vi "receive_photon_buffer.vi"(8 "error in (no error)":errorcluster, 11 "picoharp in":refnum<class "picoharp.lvclass">) -> (0 "error out":errorcluster, 2 "done":bool, 3 "picoharp out":refnum<class "picoharp.lvclass">)   [LabVIEW 2015, in "picoharp.lvclass"]
uses:
  picoharp.lvclass
  picoharp.lvclass/picoharp.ctl
  Hydraharp/hydraharp/hydraharp_fifo_queue_data.ctl
  Hydraharp/hydraharp/hydraharp_fifo_actions.ctl
  phlib.dll
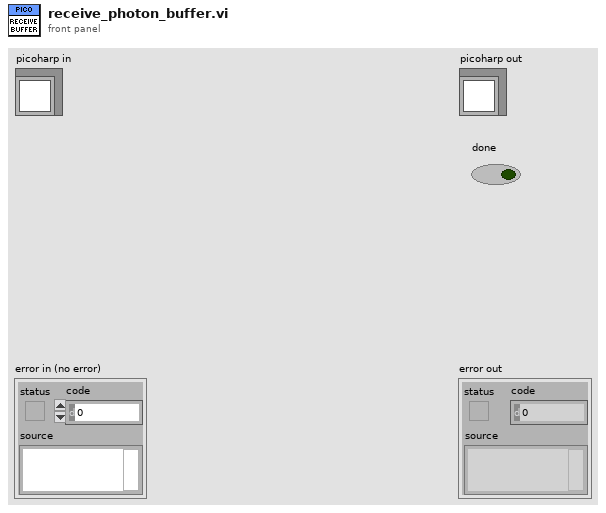
[diagram p1: front panel]
types:
  T1 = typedef "hydraharp_fifo_queue_data.ctl" = cluster{"fifo_buffer":u32[], "fifo_action":T2}
  T2 = typedef "hydraharp_fifo_actions.ctl" = enum16{"stop", "new_data"}
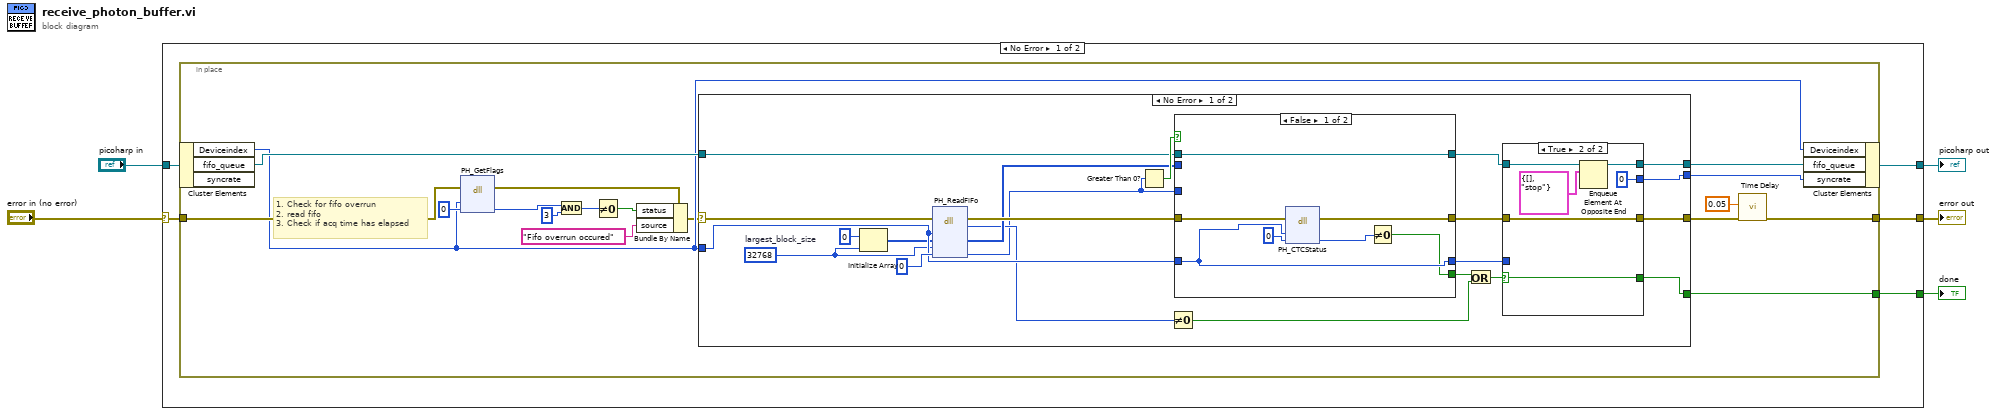
[diagram p0: block diagram]
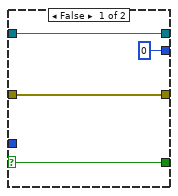
[diagram p2: hidden frame]
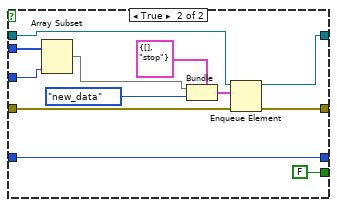
[diagram p3: hidden frame]
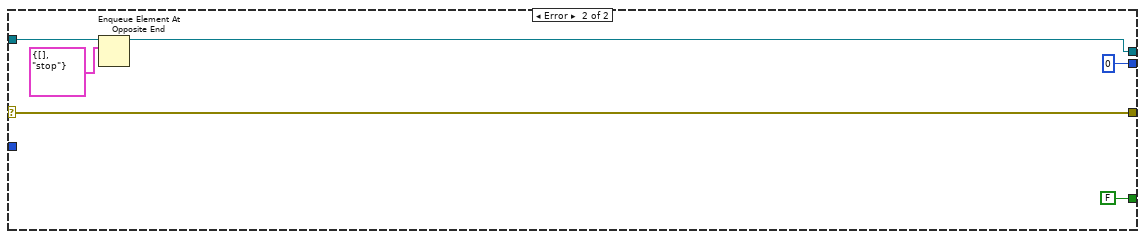
[diagram p4: hidden frame]
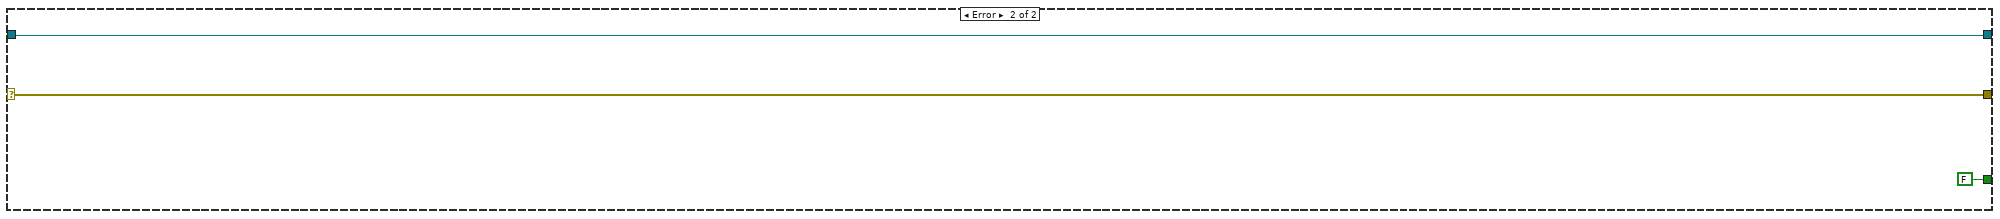
[diagram p5: hidden frame]
diagram:
  n1 = case shown="No Error" "error in (no error)" {
    selector: "error in (no error)" -> [w9 w87]
    tunnel: [w8 w87] -> w2
    tunnel: [w7 w86] -> w1
    tunnel: "picoharp in" -> [w10 w86]
    tunnel: [w6 FALSE] -> w3
    frame No Error {
      n2 = in-place {
        in-place-border: w9 -> [w27]
        in-place-border: [w12] -> w8
        in-place-border: [w20] -> w6
        # "1. Check for fifo overrun\n2. read fifo\n3. Check if acq time has elapsed"
        n3 = in-place-cluster #1(w10) -> ("Deviceindex"=w21:i32, "fifo_queue"=w23:refnum<queue>)  [unwired: 1 out]
        n4 = dll-call lib="phlib.dll" fn="PH_GetFlags" label="pH_GetFlags"(error in=w27, "devidx"=w21, "flags"=0) -> (error out=w19:errorcluster, "flags"=w25:i32)  [unwired: 4 in, 1 out]
        n5 = And(x=w25, y=3) -> (x .and. y?=w16:i32)
        n6 = Not Equal To 0?(x=w16) -> (x != 0?=w15:bool)
        n7 = Bundle By Name(cluster=w19, "status"=w15, "source"="Fifo overrun occured") -> (w17:errorcluster)
        n8 = case shown="No Error" w17 {
          selector: w17 -> [w37 w80]
          tunnel: w21 -> [w46 _]
          tunnel: w23 -> [w44 w84]
          tunnel: [w40 w83] -> w22
          tunnel: [w39 w80] -> w13
          tunnel: [w38 FALSE] -> w20
          tunnel: [w28 0 ("syncrate")] -> w11
          frame No Error {
            w31 = 32768  # largest_block_size
            n9 = Initialize Array(u32 0 ("element"), w31) -> (w30:u32[])
            n10 = dll-call lib="phlib.dll" fn="PH_ReadFiFo" label="pH_ReadFiFo"(error in=w37, "devidx"=w46, "buffer"=w30, "blocksize"=w31, "nactual"=0) -> (error out=w47:errorcluster, "return type"=w36:i32, "buffer"=w43:u32[], "nactual"=w33:i32)  [unwired: 4 in, 1 out]
            n11 = Greater Than 0?(x=w33) -> (x > 0?=w48:bool)
            n12 = Not Equal To 0?(x=w36) -> (x != 0?=w35:bool)
            n13 = case shown="False" w48 {
              tunnel: w47 -> [w66 w76]
              tunnel: [w65 w71] -> w34
              tunnel: w46 -> [w63 w67]
              tunnel: [w60 FALSE] -> w45
              tunnel: w44 -> [w64 w77]
              tunnel: w43 -> [_ w70]
              tunnel: [w64 w72] -> w41
              tunnel: w33 -> [_ w68]
              tunnel: [w63 w67] -> w29
              frame False {
                n14 = dll-call lib="phlib.dll" fn="PH_CTCStatus" label="pH_CTCStatus"(error in=w66, "devidx"=w63, "status"=0) -> (error out=w65:errorcluster, "status"=w61:i32)  [unwired: 4 in, 1 out]
                n15 = Not Equal To 0?(x=w61) -> (x != 0?=w60:bool)
              }
              frame True {
                n16 = Array Subset(array=w70, length=w68) -> (w69:u32[])  [unwired: 1 in]
                n17 = Bundle(cluster=T1 {"fifo_buffer"=[], "fifo_action"=enum."stop"} ("output cluster"), "fifo_buffer"=w69, "fifo_action"=hydraharp_fifo_actions."new_data") -> (w73:T1)
                n18 = Enqueue Element(queue=w77, element=w73, error in (no error)=w76) -> (queue out=w72:refnum<queue>, error out=w71:errorcluster)  [unwired: 1 in, 1 out]
              }
            }
            n19 = Or(x=w45, y=w35) -> (x .or. y?=w42:bool)
            n20 = case shown="True" w42 {
              selector: w42 -> [w51 w56]
              tunnel: w41 -> [w53 w59]
              tunnel: [w53 w57] -> w40
              tunnel: w34 -> [w52 w55]
              tunnel: [w52 w55] -> w39
              tunnel: [w51 w56] -> w38
              tunnel: w29 -> [_ _]
              tunnel: [0 ("syncrate") 0 ("syncrate")] -> w28
              frame False {
              }
              frame True {
                n21 = Enqueue Element At Opposite End(queue=w59, element=T1 {"fifo_buffer"=[], "fifo_action"=enum."stop"}) -> (queue out=w57:refnum<queue>)  [unwired: 2 in, 2 out]
              }
            }
          }
          frame Error {
            n22 = Enqueue Element At Opposite End(queue=w84, element=T1 {"fifo_buffer"=[], "fifo_action"=enum."stop"}) -> (queue out=w83:refnum<queue>)  [unwired: 2 in, 2 out]
          }
        }
        n23 = call "Time Delay"("error in (no error)"=w13, "Delay Time (s)"=0.05) -> ("error out"=w12:errorcluster)  [unwired: 9 in]
        n24 = in-place-cluster #1("Deviceindex"=w21, "fifo_queue"=w22, "syncrate"=w11) -> (w7:refnum<class "picoharp.lvclass">)
      }
    }
    frame Error {
    }
  }
  "error out" <- w2
  "picoharp out" <- w1
  "done" <- w3
